vi "Main - Page eFGV.vi"(7 "eFGV States":T2, 8 "error in (no error)":errorcluster, 11 "Page In":T1(ring)) -> (0 "error out":errorcluster, 2 "Page ref":refnum<user-event>, 3 "Page Out":T1(ring))   [LabVIEW 2019]
doc: "event FGV where it will trigger to stop all the process in the program"
uses:
  Controls/eFGV States.ctl
  <vilib>/event_ctls.llb/usereventprio.ctl
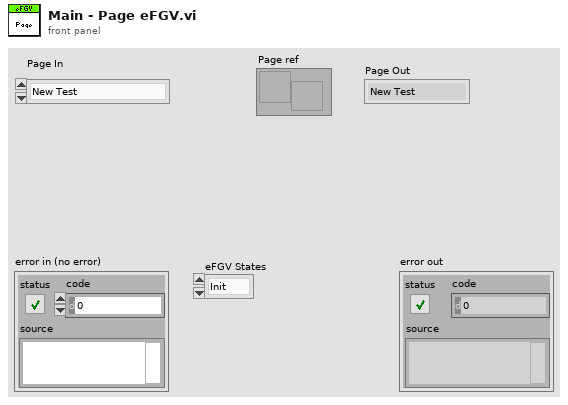
[diagram p1: front panel]
types:
  T1 = enum16{"New Test", "Test Plan", "Job Record", "Instrument", "Machine", "Station", "Machine Control"}
  T2 = typedef "eFGV States.ctl" = enum16{"Init", "Read", "Write", "Exit"}
  T3 = typedef "usereventprio.ctl" = enum32{"high priority", "normal priority"}
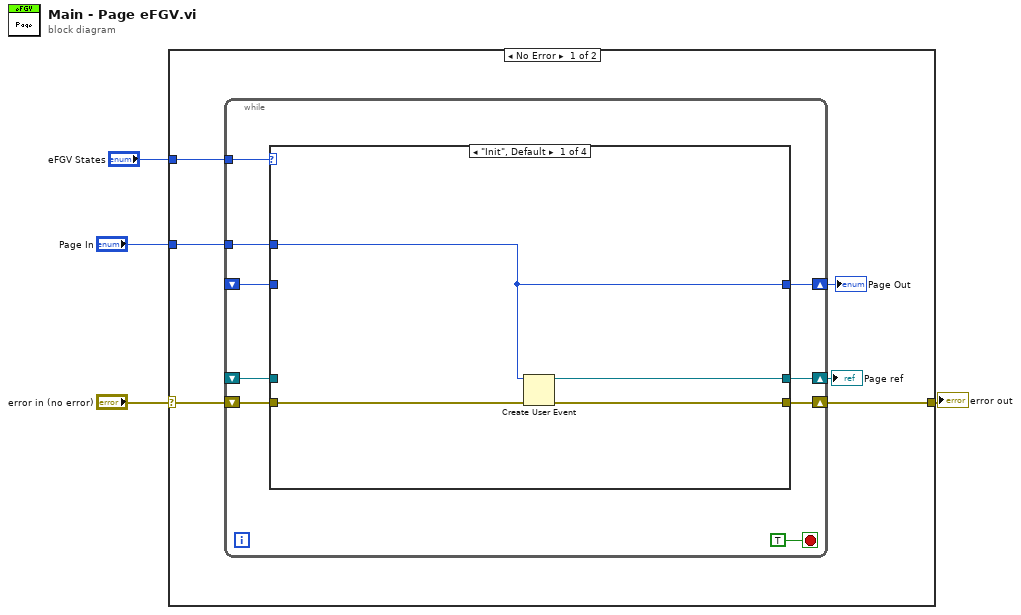
[diagram p0: block diagram]
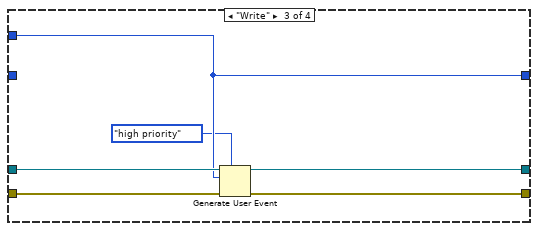
[diagram p3: hidden frame]
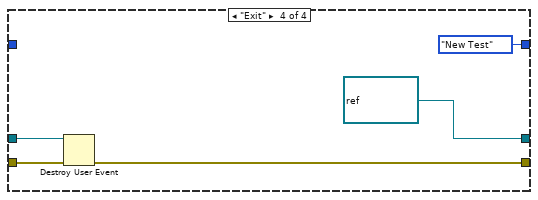
[diagram p4: hidden frame]
diagram:
  n1 = case shown="No Error" "error in (no error)" {
    selector: "error in (no error)" -> [w9 w38]
    tunnel: "eFGV States" -> [w10 _]
    tunnel: "Page In" -> [w8 _]
    tunnel: [w7 w38] -> w1
    frame No Error {
      n2 = while {
        tunnel: w10 -> [w18]
        shift-right: [w15] -> w7
        shift-left: w9 -> [w17]
        tunnel: w8 -> [w16]
        shift-right: [w14] -> w5
        shift-left: _ -> [w13]
        shift-right: [w12] -> w6
        shift-left: _ -> [w11]
        stop <- TRUE stop-if-true
        n3 = case shown="\"Init\", Default" w18 {
          tunnel: w17 -> [w23 w25 w30 w37]
          tunnel: w16 -> [w21 _ w29 _]
          tunnel: [w22 w25 w31 w35] -> w15
          tunnel: [w21 w26 w29 T1."New Test" ("Page In")] -> w14
          tunnel: w13 -> [_ w26 _ _]
          tunnel: w11 -> [_ w24 w32 w36]
          tunnel: [w20 w24 w27 w34] -> w12
          frame "Init", Default {
            n4 = Create User Event(user event datatype=w21, error in=w23) -> (user event=w20:refnum<user-event>, error out=w22:errorcluster)
          }
          frame "Read" {
          }
          frame "Write" {
            n5 = Generate User Event(priority (normal)=usereventprio."high priority", user event=w32, event data cluster=w29, error in=w30) -> (user event out=w27:refnum<user-event>, error out=w31:errorcluster)
          }
          frame "Exit" {
            w34 = refnum<user-event> refnum items=["New Test", "Test Plan", "Job Record", "Instrument", "Machine", "Station", "Machine Control"] ("Page In")
            n6 = Destroy User Event(user event=w36, error in=w37) -> (error out=w35:errorcluster)
          }
        }
      }
      "Page ref" <- w6
      "Page Out" <- w5
    }
    frame Error {
    }
  }
  "error out" <- w1
